vi "AvrgSGL.vi"(4 "b":sgl, 5 "a":sgl) -> (1 "Average of a and b":sgl)   [LabVIEW 2017, in "GPNumeric.lvlib"]
doc: "Calculates the average value of <B>a</B> and <B>b</B>.\n\nThis VI is inlined.\n\nSteen Schmidt\nGPower\n24/11 2014"
uses:
  GPNumeric.lvlib
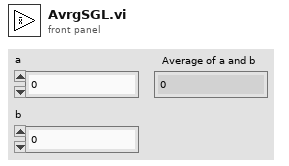
[diagram p1: front panel]
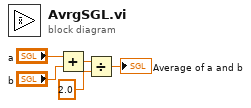
[diagram p0: block diagram]
diagram:
  n1 = Add(x="a", y="b") -> (x+y=w3:sgl)
  n2 = Divide(x=w3, y=sgl 2.0) -> (x/y=→"Average of a and b":sgl)
